vi "Reset Abort.vi"(8 "error in (no error)":errorcluster, 11 "AbortHandler in":refnum<class "Abortable.lvclass">) -> (0 "error out":errorcluster, 3 "AbortHandler out":refnum<class "Abortable.lvclass">)   [LabVIEW 2020, in "Volatus.lvlib" / "Abortable.lvclass"]
uses:
  Abortable.lvclass
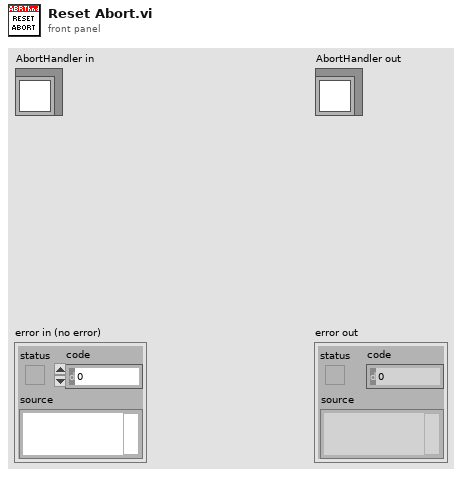
[diagram p1: front panel]
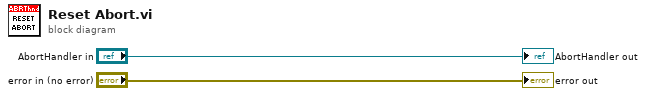
[diagram p0: block diagram]
diagram:
  "error out" <- "error in (no error)"
  "AbortHandler out" <- "AbortHandler in"
